vi "libssh2_channel_setenv_ex.vi"(8 "error in (no error)":errorcluster, 9 "value":string, 10 "varname":string, 11 "channel":T1) -> (0 "error out":errorcluster)   [LabVIEW 2017, in "libssh2.lvlib"]
doc: "Set an environment variable on a channel."
uses:
  libssh2.lvlib
  Channel Refnum.ctl
  Acquire Session.vi
  Release Session.vi
  Not A Channel.vi
  <vilib>/Utility/error.llb/Error Cluster From Error Code.vi
  Global Settings.vi
  Read Channel Refnum.vi
  Read Session Refnum.vi
  <vilib>/Utility/semaphor.llb/Acquire Semaphore.vi
  <vilib>/Utility/semaphor.llb/Release Semaphore.vi
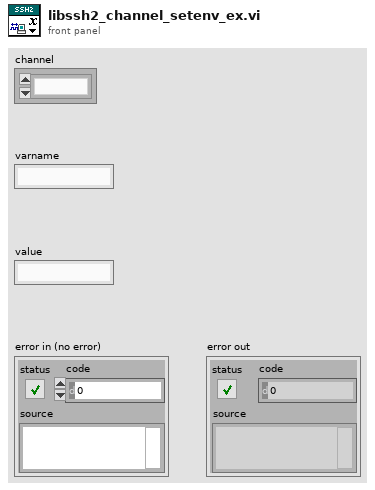
[diagram p1: front panel]
types:
  T1 = typedef "libssh2.lvlib/Channel Refnum.ctl" = refnum<k1>
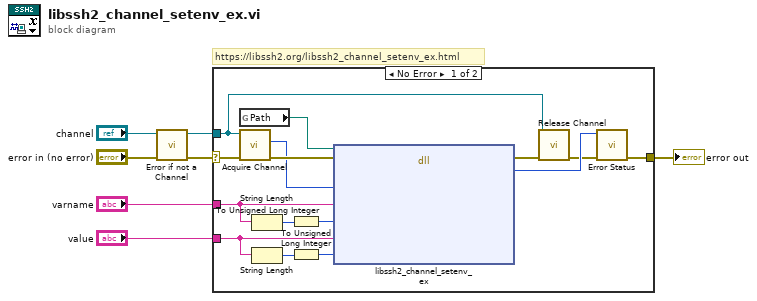
[diagram p0: block diagram]
diagram:
  # "https://libssh2.org/libssh2_channel_setenv_ex.html"
  n1 = call "Error if not a Channel.vi"("error in (no error)"="error in (no error)", "channel"="channel") -> ("error out"=w5:errorcluster, "channel out"=w3:T1)  [unwired: 8 in]
  n2 = case shown="No Error" w5 {
    selector: w5 -> [w21 w23]
    tunnel: [w11 w23] -> w7
    tunnel: w3 -> [w8 _]
    tunnel: "varname" -> [w17 _]
    tunnel: "value" -> [w13 _]
    frame No Error {
      n3 = global read "Global Settings.vi" "Path"() -> (w18:path)
      n4 = call "Acquire Channel.vi"("error in (no error)"=w21, "channel"=w8) -> ("error out"=w20:errorcluster, "LIBSSH2_CHANNEL*"=w19:u64)  [unwired: 8 in]
      n5 = String Length(string=w17) -> (length=w16:i32)
      n6 = String Length(string=w13) -> (length=w14:i32)
      n7 = To Unsigned Long Integer(number=w16) -> (unsigned 32bit integer=w15:u32)
      n8 = To Unsigned Long Integer(number=w14) -> (unsigned 32bit integer=w12:u32)
      n9 = dll-call lib="?" fn="libssh2_channel_setenv_ex"(path in=w18, error in=w20, "channel"=w19, "varname"=w17, "varname_len"=w15, "value"=w13, "value_len"=w12) -> (error out=w22:errorcluster, "return value"=w10:i32)  [unwired: 6 in, 1 out]
      n10 = call "Release Channel.vi"("error in (no error)"=w22, "channel"=w8) -> ("error out"=w9:errorcluster)  [unwired: 9 in]
      n11 = call "Error Status.vi"("error in (no error)"=w9, "return value"=w10) -> ("error out"=w11:errorcluster)  [unwired: 8 in, 1 out]
    }
    frame Error {
    }
  }
  "error out" <- w7
